vi "medidorIXV.vi"(7 "Ponto":i32) -> (1 "Array":dbl[](array[numeric]), 2 "Corrente Atual":dbl, 3 "Tensao Atual":dbl)   [LabVIEW 2012]
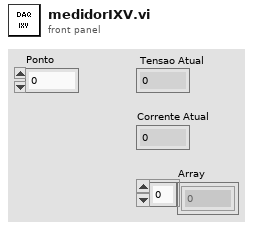
[diagram p1: front panel]
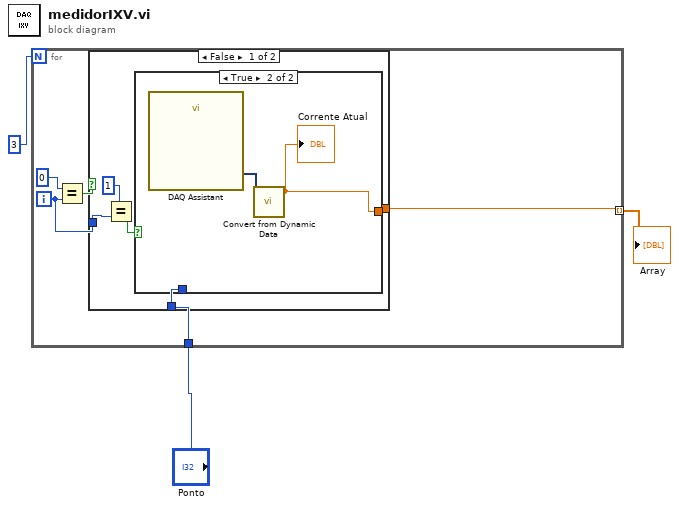
[diagram p0: block diagram]
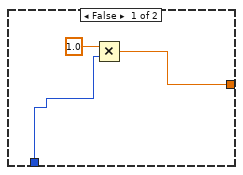
[diagram p2: hidden frame]
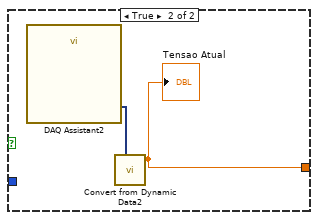
[diagram p3: hidden frame]
diagram:
  n1 = for {
    N: 3 -> [_]
    tunnel: [w5] -> w1 mode=indexing
    tunnel: "Ponto" -> [w4]
    i -> [w6]
    n2 = Equal?(x=0, y=w6) -> (x = y?=w7:bool)
    n3 = case shown="False" w7 {
      tunnel: [w9 w19] -> w5
      tunnel: w6 -> [w12 _]
      tunnel: w4 -> [w10 _]
      frame False {
        n4 = Equal?(x=1, y=w12) -> (x = y?=w11:bool)
        n5 = case shown="True" w11 {
          tunnel: w10 -> [w14 _]
          tunnel: [w16 w17] -> w9
          frame False {
            n6 = Multiply(x=1.0, y=w14) -> (x*y=w16:dbl)
          }
          frame True {
            n7 = call "DAQ Assistant"() -> ("data"=w18:dynamicdata)  [unwired: 17 in, 2 out]
            n8 = call "Convert from Dynamic Data"("Dynamic Data Type"=w18) -> ("Scalar"=w17:dbl)  [unwired: 3 in]
            "Corrente Atual" <- w17
          }
        }
      }
      frame True {
        n9 = call "DAQ Assistant2"() -> ("data"=w20:dynamicdata)  [unwired: 17 in, 2 out]
        n10 = call "Convert from Dynamic Data2"("Dynamic Data Type"=w20) -> ("Scalar"=w19:dbl)  [unwired: 3 in]
        "Tensao Atual" <- w19
      }
    }
  }
  "Array" <- w1
